vi "TFG_Rev0.vi"() -> ()   [LabVIEW 2019]
uses:
  <vilib>/Instr/_visa.llb/VISA Configure Serial Port (Instr).vi
  VARIABLES_GLOBAL.vi
panel:
  out "PH":dbl
  out "concatenated string":string
  out "TEMPERATURA":dbl(knob) scale=0.0..50.0
  out "HUMEDAD":dbl(knob) scale=0.0..100.0
  out "TEMPERATURA":dbl
  out "HUMEDAD RELATIVA":dbl
  in  "Introdución de parámetros":bool
  out "ASPERSOR":bool
  in  "FUNCIONAMIENTO MANUAL":bool
  in  "ASPERSOR":bool
  out "PH+":bool
  out "PH-":bool
  in  "RIEGO":bool
  in  "PH-":bool
  out "CALEFACTOR":bool
  out "VENTANA":bool
  out "RIEGO":bool
  in  "PH+":bool
  in  "CALEFACTOR":bool
  in  "VENTANA":bool
  out "PH":dbl(knob) scale=0.0..14.0
  in  "Selección de vivero":refnum<visa-resource-name>
  # "Rubén Garrido - Universitat de València E.T.S.E"
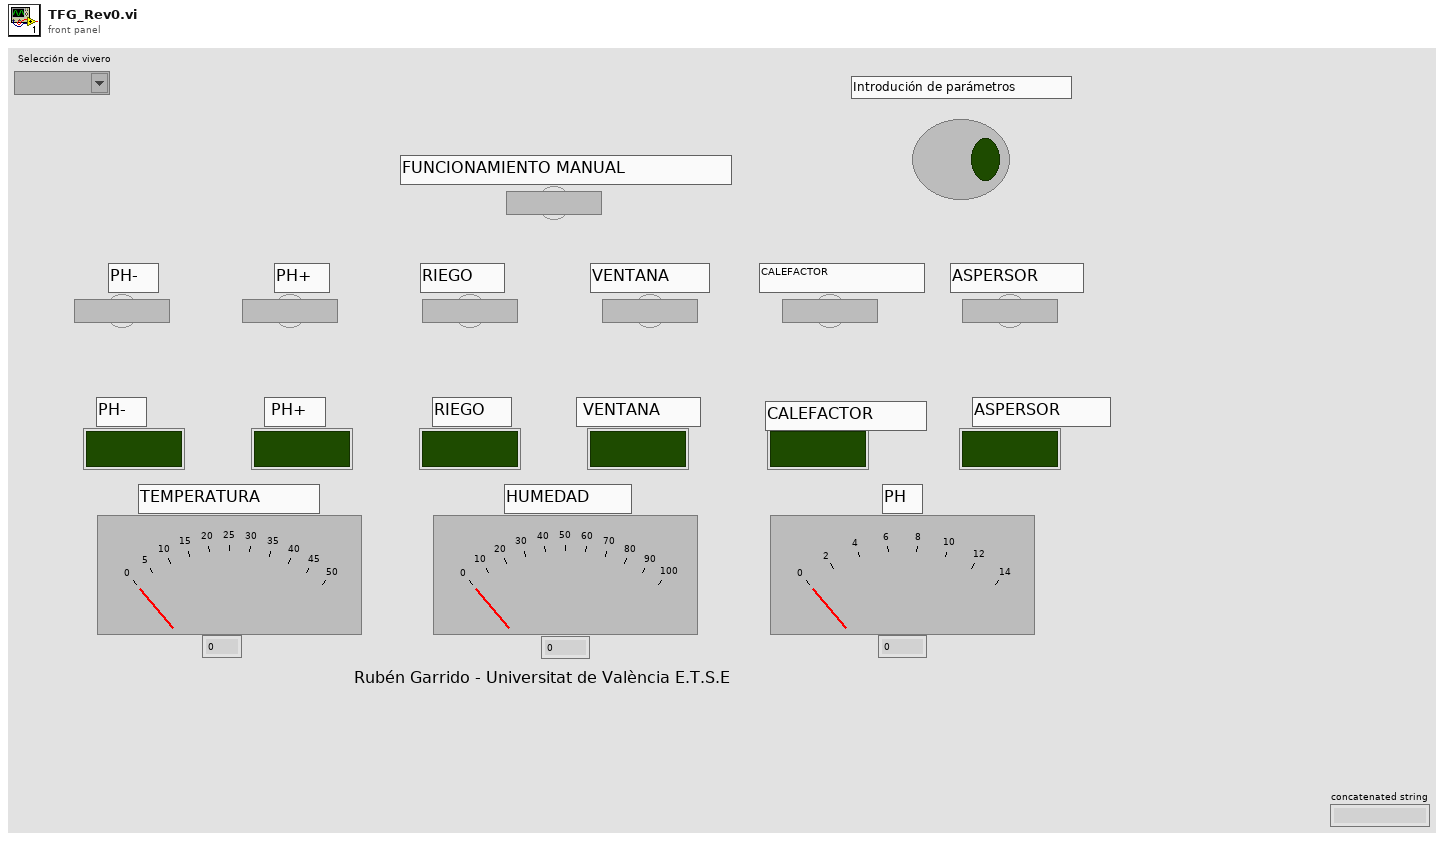
[diagram p1: front panel]
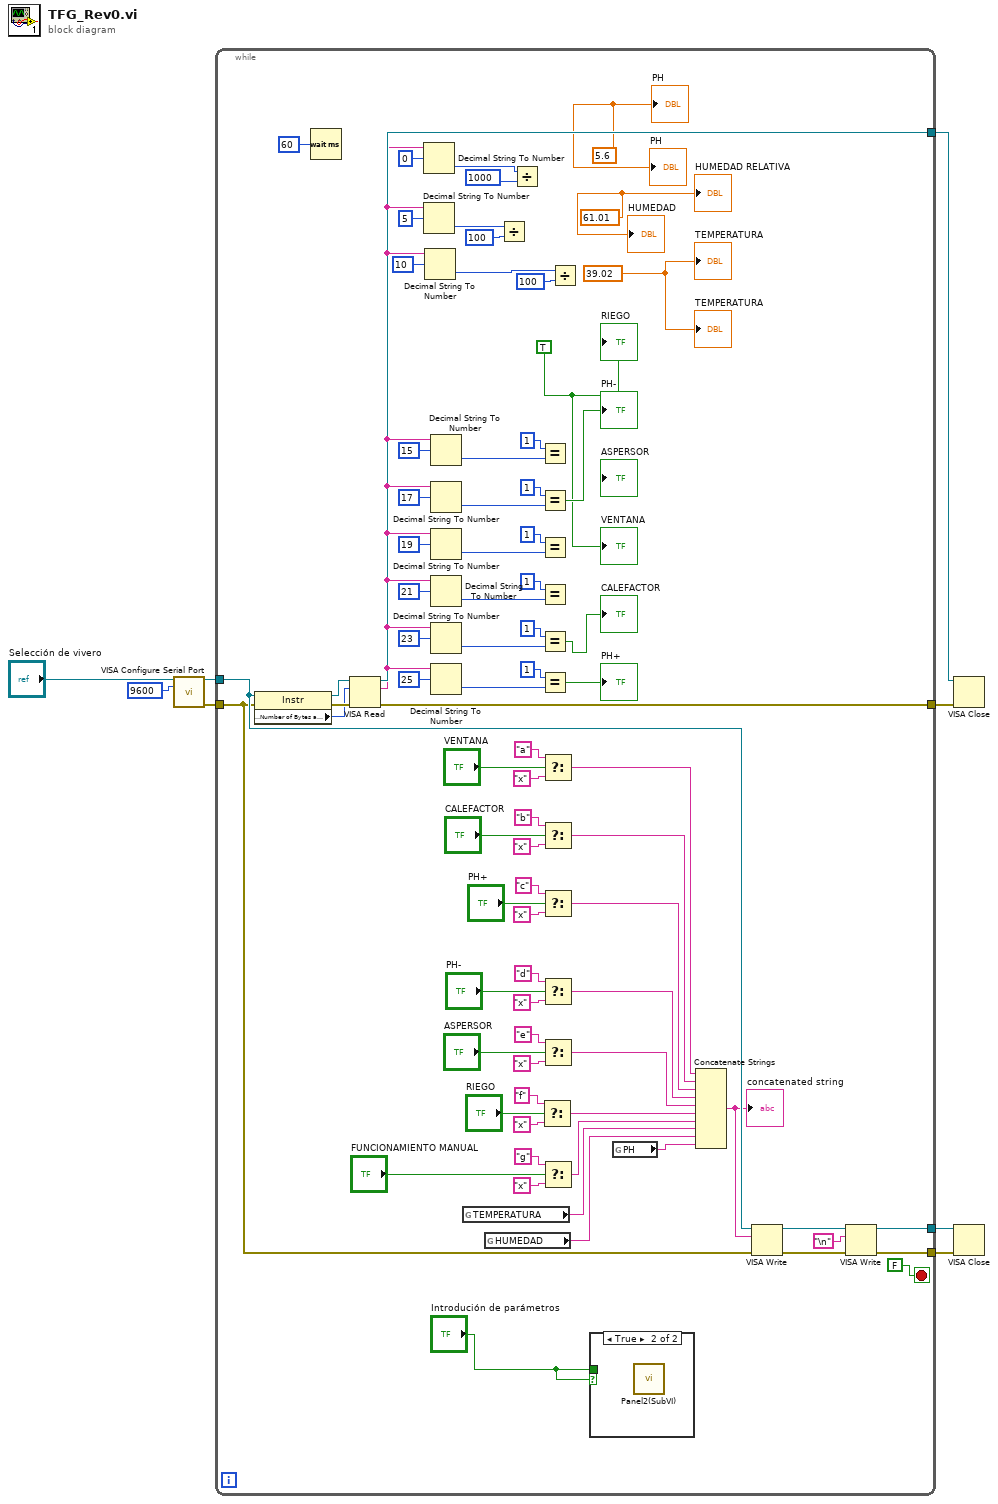
[diagram p0: block diagram]
diagram:
  n1 = call-poly "VISA Configure Serial Port"("VISA resource name"="Selección de vivero", "baud rate (9600)"=u32 9600) -> ("VISA resource name out"=w8:refnum<visa-resource-name>, "error out"=w7:errorcluster)  [unwired: 12 in]
  n2 = while {
    tunnel: w8 -> [w68]
    tunnel: w7 -> [w67]
    tunnel: [w72] -> w4
    tunnel: [w71] -> w3
    tunnel: [w70] -> w2
    tunnel: [w69] -> w1
    stop <- FALSE stop-if-true
    w9 = 39.02 ("TEMPERATURA")
    w10 = 61.01 ("HUMEDAD RELATIVA")
    w11 = 5.6 ("PH")
    w12 = TRUE ("RIEGO")
    n3 = property class="Instr"(reference=w68, error in=w67) -> (reference out=w90:refnum<visa-resource-name>, error out=w89:errorcluster, "Serial Settings:Number of Bytes at Serial Port"=w88:u32)
    n4 = Wait (ms)(milliseconds to wait=u32 60) -> ()  [unwired: 1 out]
    n5 = VISA Read(VISA resource name=w90, byte count=w88, error in (no error)=w89) -> (VISA resource name out=w70:refnum<visa-resource-name>, read buffer=w30:string, error out=w69:errorcluster)  [unwired: 1 out]
    n6 = Decimal String To Number(string=w30, offset=0) -> (number=w15:i32)  [unwired: 1 in, 1 out]
    n7 = Decimal String To Number(string=w30, offset=5) -> (number=w20:i32)  [unwired: 1 in, 1 out]
    n8 = Decimal String To Number(string=w30, offset=10) -> (number=w18:i32)  [unwired: 1 in, 1 out]
    n9 = Decimal String To Number(string=w30, offset=15 ("offset (0)")) -> (number=w63:i32)  [unwired: 1 in, 1 out]
    n10 = Decimal String To Number(string=w30, offset=17 ("offset (0)")) -> (number=w43:i32)  [unwired: 1 in, 1 out]
    n11 = Decimal String To Number(string=w30, offset=19 ("offset (0)")) -> (number=w31:i32)  [unwired: 1 in, 1 out]
    n12 = Decimal String To Number(string=w30, offset=21 ("offset (0)")) -> (number=w59:i32)  [unwired: 1 in, 1 out]
    n13 = Decimal String To Number(string=w30, offset=23 ("offset (0)")) -> (number=w57:i32)  [unwired: 1 in, 1 out]
    n14 = Decimal String To Number(string=w30, offset=25 ("offset (0)")) -> (number=w45:i32)  [unwired: 1 in, 1 out]
    n15 = global read "VARIABLES_GLOBAL.vi" "TEMPERATURA"() -> (w23:string)
    n16 = global read "VARIABLES_GLOBAL.vi" "HUMEDAD"() -> (w22:string)
    n17 = Divide(x=w20, y=100) -> ()  [unwired: 1 out]
    n18 = Divide(x=w15, y=1000) -> ()  [unwired: 1 out]
    n19 = Equal?(x=1 ("y"), y=w63) -> ()  [unwired: 1 out]
    n20 = Equal?(x=1 ("y"), y=w43) -> (x = y?=→"PH-":bool)
    n21 = Equal?(x=1 ("y"), y=w31) -> ()  [unwired: 1 out]
    n22 = Equal?(x=1 ("y"), y=w59) -> ()  [unwired: 1 out]
    n23 = Equal?(x=1 ("y"), y=w57) -> (x = y?=→"CALEFACTOR":bool)
    n24 = Equal?(x=1 ("y"), y=w45) -> (x = y?=→"PH+":bool)
    n25 = Select(t="f", s="RIEGO", f="x") -> (s? t:f=w34:string)
    n26 = Select(t="a", s="VENTANA", f="x") -> (s? t:f=w29:string)
    n27 = Select(t="b", s="CALEFACTOR", f="x") -> (s? t:f=w28:string)
    n28 = Select(t="c", s="PH+", f="x") -> (s? t:f=w27:string)
    n29 = Select(t="d", s="PH-", f="x") -> (s? t:f=w25:string)
    n30 = Select(t="e", s="ASPERSOR", f="x") -> (s? t:f=w26:string)
    n31 = Select(t="g", s="FUNCIONAMIENTO MANUAL", f="x") -> (s? t:f=w24:string)
    n32 = Divide(x=w18, y=100) -> ()  [unwired: 1 out]
    n33 = case shown="True" "Introdución de parámetros" {
      tunnel: "Introdución de parámetros" -> [_ _]
      frame False {
      }
      frame True {
        n34 = call "Panel2(SubVI).vi"() -> ()  [unwired: 12 in]
      }
    }
    n35 = global read "VARIABLES_GLOBAL.vi" "PH"() -> (w21:string)
    n36 = Concatenate Strings(w29, w28, w27, w25, w26, w34, w24, w23, w22, w21) -> (w66:string)
    "concatenated string" <- w66
    n37 = VISA Write(VISA resource name=w68, write buffer=w66, error in (no error)=w67) -> (VISA resource name out=w84:refnum<visa-resource-name>, error out=w83:errorcluster)  [unwired: 1 out]
    n38 = VISA Write(VISA resource name=w84, write buffer="\n", error in (no error)=w83) -> (VISA resource name out=w72:refnum<visa-resource-name>, error out=w71:errorcluster)  [unwired: 1 out]
    "PH" <- w11
    "VENTANA" <- w12
    "RIEGO" <- w12
    "HUMEDAD RELATIVA" <- w10
    "TEMPERATURA" <- w9
    "HUMEDAD" <- w10
    "TEMPERATURA" <- w9
    "PH" <- w11
  }
  n39 = VISA Close(VISA resource name=w2, error in (no error)=w1) -> ()  [unwired: 1 out]
  n40 = VISA Close(VISA resource name=w4, error in (no error)=w3) -> ()  [unwired: 1 out]
